vi "GETCursor.vi"(7 "LabVIEW Web Service Request":refnum<class "Web Request.lvclass">) -> (3 "LabVIEW Web Service Request out":refnum<class "Web Request.lvclass">)   [LabVIEW 2014]
uses:
  <vilib>/wsapi/Web Request.lvclass
  Libraries/Map Data Folder/Map Data.lvlib
panel:
  # "Use the Web Service Request input terminal to call the VIs on the Web Services palette. Do not remove it from the connector pane unless you don't need access to the palette."
  # "Each additional control wired to the connector pane will be available as an input in the URL. To include an indicator in terminal-mode output (the default setting), it must also be wired to the connector pane."
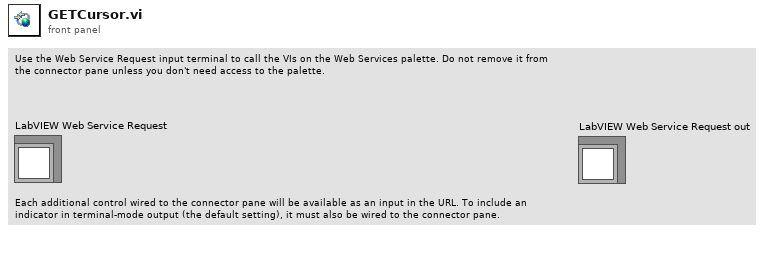
[diagram p1: front panel]
types:
  T1 = typedef "Map Data.lvlib/CursorList.ctl" = cluster{"Name":string, "Color":u32, "Style":u8, "Point Style":u8, "Name Visible":bool, "Allow Drag":bool, "Cursor Mode":u32, "Plot":i32, "Index":i32, "Position":cluster{"X":dbl, "Y":dbl}, "X Scale":u32, "Y Scale":u32, "Watch Plots":i32[], "Watch All Plots":bool, "Plot Area":i32, "Label Offset":cluster{"X":dbl, "Y":dbl}}[]
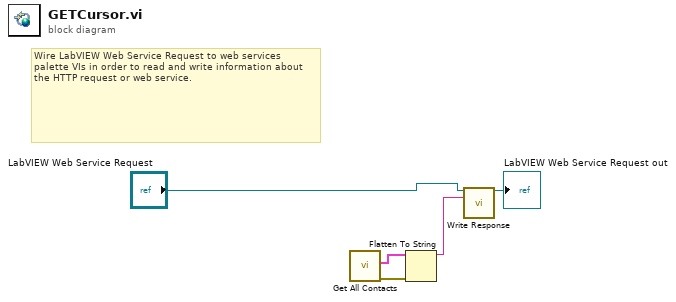
[diagram p0: block diagram]
diagram:
  # "Wire LabVIEW Web Service Request to web services palette VIs in order to read and write information about the HTTP request or web service."
  n1 = call "Get All Contacts.vi"() -> ("error out"=w5:errorcluster, "Cursor List"=w1:T1)  [unwired: 9 in, 1 out]
  n2 = Flatten To String(anything=w1, error in (no error)=w5) -> (data string=w3:string)  [unwired: 2 in, 2 out]
  n3 = call <vilib>:"Write Response.vi"("LabVIEW Web Service Request"="LabVIEW Web Service Request", "response string"=w3) -> ("LabVIEW Web Service Request out"=→"LabVIEW Web Service Request out":refnum<class "Web Request.lvclass">)  [unwired: 12 in, 1 out]
